vi "SetVelocitySetpointXaxis.vi"(10 "Xaxis":dbl, 11 "DriveBase.lvclass":refnum<class "DriveBase.lvclass">) -> (3 "DriveBase.lvclass":refnum<class "DriveBase.lvclass">)   [LabVIEW 2016, in "DriveBase.lvclass"]
uses:
  DriveBase.lvclass
  DriveBase.lvclass/DriveBase.ctl
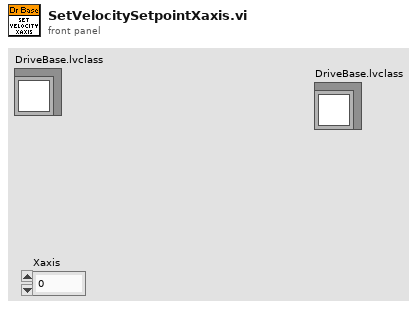
[diagram p1: front panel]
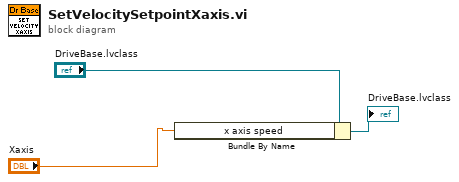
[diagram p0: block diagram]
diagram:
  n1 = Bundle By Name(cluster="DriveBase.lvclass", "x axis speed"="Xaxis") -> (→"DriveBase.lvclass":refnum<class "DriveBase.lvclass">)
